vi "I2C Read Byte.vi"(8 "error in (no error)":errorcluster, 10 "Address":u8 format="%.0x", 11 "LINX-PCA9865 PWM in":refnum<class "LINX-PCA9865 PWM.lvclass">) -> (0 "error out":errorcluster, 2 "Byte Read":u8, 3 "LINX-PCA9865 PWM out":refnum<class "LINX-PCA9865 PWM.lvclass">)   [LabVIEW 2019, in "LINX-PCA9865 PWM.lvclass"]
uses:
  LINX-PCA9865 PWM.lvclass
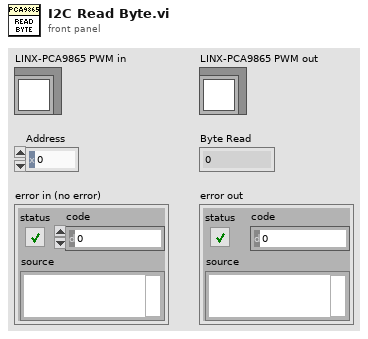
[diagram p1: front panel]
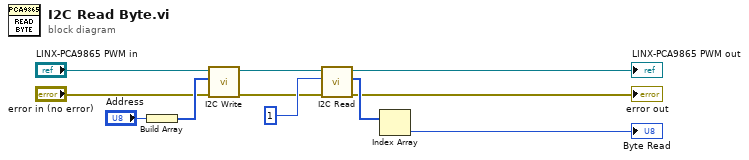
[diagram p0: block diagram]
diagram:
  n1 = Build Array("Address") -> (w11:u8[])
  n2 = call "I2C Write.vi"("error in (no error)"="error in (no error)", "Bytes to Write"=w11, "LINX-PCA9865 PWM in"="LINX-PCA9865 PWM in") -> ("error out"=w5:errorcluster, "LINX-PCA9865 PWM out"=w3:refnum<class "LINX-PCA9865 PWM.lvclass">)  [unwired: 7 in]
  n3 = call "I2C Read.vi"("error in (no error)"=w5, "# Bytes to Read"=u8 1, "LINX-PCA9865 PWM in"=w3) -> ("error out"=→"error out":errorcluster, "Bytes Read"=w8:u8[], "LINX-PCA9865 PWM out"=→"LINX-PCA9865 PWM out":refnum<class "LINX-PCA9865 PWM.lvclass">)  [unwired: 6 in]
  n4 = Index Array(array=w8) -> (element=→"Byte Read":u8)  [unwired: 1 in]
